vi "2DHistogram.vi"() -> ()   [LabVIEW 2022 SP3]
uses:
  <vilib>/Utility/file.llb/Read From Spreadsheet File (DBL).vi
  <vilib>/Utility/file.llb/Write To Spreadsheet File (I64).vi
panel:
  out "size in":i32
  out "mid min value":sgl format="%.2f"
  out "mid max value":sgl format="%.2f"
  out "int min value":sgl format="%.2f"
  out "int max value":sgl format="%.2f"
  in  "Grid Size":i32=5
  out "total pts":i32
  in  "Save file?":bool
  out "Array":i32[][](array[numeric])
  out "Midband":dbl[](array[numeric]) format="%.2f"
  out "Int":dbl[](array[numeric]) format="%.2f"
  # "INPUT FILE NEEDS INTERCEPT VALUES COLUMN ONE AND MIDBAND IN COLUMN TWO IN SPREADSHEET FORMAT. ROWS ARE MIDBANDINTERCEPT AND COLUMNS  INTERCEPT IN OUTPUT FILE"
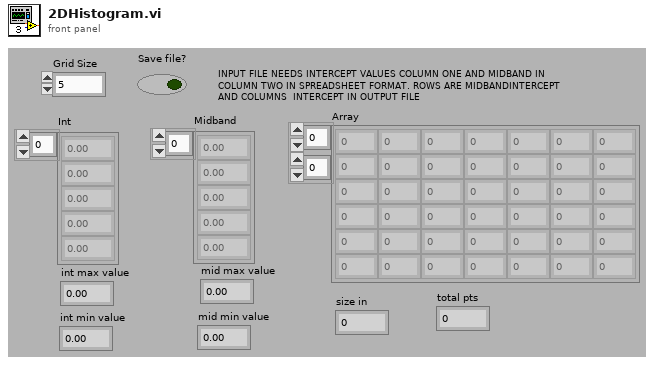
[diagram p1: front panel]
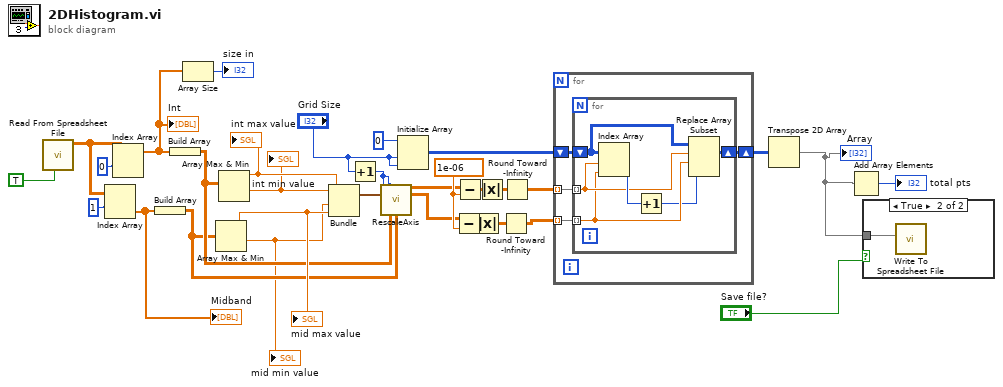
[diagram p0: block diagram]
diagram:
  w11 = 1e-06
  n1 = call-poly <vilib>:"Read From Spreadsheet File.vi"("transpose (no:F)"=TRUE) -> ("all rows"=w25:dbl[][])  [unwired: 3 in, 7 out]
  n2 = Index Array(array=w25, index (row)=1) -> (element=w2:dbl[])  [unwired: 1 in]
  "Midband" <- w2
  n3 = Index Array(array=w25, index (row)=0) -> (element=w3:dbl[])  [unwired: 1 in]
  "Int" <- w3
  n4 = Build Array(w2) -> (w21:dbl[][])
  n5 = Build Array(w3) -> (w22:dbl[][])
  n6 = Array Size(array=w3) -> (size(s)=→"size in":i32)
  n7 = Array Max & Min(array=w21) -> (max value=w29:dbl, min value=w14:dbl)  [unwired: 2 out]
  "mid max value" <- w29
  "mid min value" <- w14
  n8 = Array Max & Min(array=w22) -> (max value=w30:dbl, min value=w15:dbl)  [unwired: 2 out]
  "int max value" <- w30
  "int min value" <- w15
  n9 = Bundle(w30, w15, w14, w29) -> (w31:cluster{dbl, dbl, dbl, dbl})  [unwired: 1 out]
  n10 = Increment(x="Grid Size") -> (x+1=w16:i32)
  n11 = call "RescaleAxis.vi"("pixels in x"=w16, "pixels in y"=w16, "Axis scaling Params"=w31, "x"=w22, "y"=w21) -> ("x scaled"=w5:dbl[][], "y scaled"=w4:dbl[][])  [unwired: 9 out]
  n12 = Initialize Array(0, "Grid Size", "Grid Size") -> (w27:i32[][])
  n13 = Subtract(x=w4, y=w11) -> (x-y=w12:dbl[][])
  n14 = Subtract(x=w5, y=w11) -> (x-y=w13:dbl[][])
  n15 = Absolute Value(x=w12) -> (abs(x)=w9:dbl[][])
  n16 = Absolute Value(x=w13) -> (abs(x)=w10:dbl[][])
  n17 = Round Toward -Infinity(1:w9) -> (0:w7:dbl[][])
  n18 = Round Toward -Infinity(1:w10) -> (0:w8:dbl[][])
  n19 = for {
    tunnel: w8 -> [w35] mode=indexing
    tunnel: w7 -> [w34] mode=indexing
    shift-right: [w32] -> w19
    shift-left: w27 -> [w33]
    n20 = for {
      tunnel: w35 -> [w40] mode=indexing
      tunnel: w34 -> [w37] mode=indexing
      shift-right: [w38] -> w32
      shift-left: w33 -> [w39]
      n21 = Index Array(array=w39, index (row)=w40, index (col)=w37) -> (element=w41:i32)
      n22 = Increment(x=w41) -> (x+1=w36:i32)
      n23 = Replace Array Subset(array=w39, new element=w36, index (row)=w40, index (col)=w37) -> (w38:i32[][])
    }
  }
  n24 = Transpose 2D Array(2D array=w19) -> (transposed array=w1:i32[][])
  "Array" <- w1
  n25 = Add Array Elements(numeric array=w1) -> (sum=→"total pts":i32)
  n26 = case shown="True" "Save file?" {
    tunnel: w1 -> [_ w42]
    frame False {
    }
    frame True {
      n27 = call-poly <vilib>:"Write To Spreadsheet File.vi"("2D data"=w42) -> ()  [unwired: 5 in, 3 out]
    }
  }
